vi "Copy Graph to Clipboard.vi"(8 "error in (no error)":errorcluster, 11 "Graph Data":T1={"UI References"={"Exit Ref"=refnum, "Save Ref"=refnum, "Open Ref"=refnum, "Export Ref"=refnum, "Acquire Ref"=refnum, "Configure Ref"=refnum, "Graph Ref"=refnum, "Clear Ref"=refnum, "Analyze Ref"=refnum, "Status Ref"=refnum, "Snapshot Ref"=refnum}, "User Specified"={"Hardware Configuration"={"VGC50"={"serial settings"={"port"="", "baud rate"=115200}, "device information"={"type"="", "model number"="", "serial number"="", "firmware version"="", "hardware version"=""}, "gauges"=[], "VGC"=refnum, "Backing SP"={"mode"=0, "thresholds"={"lower"=0.0, "upper"=0.0}, "on"=FALSE}, "Chamber SP"={"mode"=1, "thresholds"={"lower"=0.0, "upper"=0.0}, "on"=FALSE}}, "PTC10"={"serial settings"={"port"="GPIB0::22::INSTR", "baud rate"=115200}, "PTC10 Info"={"Manufacturer"="", "Instrument"="", "Serial Number"="", "Firmware"=""}, "VISA resource name"=""}}, "New Data Behavior"=enum."Replace", "Vacuum Graph config"={"Log/Lin"=FALSE, "Show Backing"=FALSE, "Show Chamber"=FALSE}}} {"User Specified"."Hardware Configuration"."PTC10"."serial settings"."baud rate" items=["9600"=9600, "19200"=19200, "38400"=38400, "57600"=57600, "115200"=115200]; "User Specified"."Hardware Configuration"."VGC50"."Chamber SP"."thresholds"."upper" format="%#_5p"; "User Specified"."Hardware Configuration"."VGC50"."Chamber SP"."thresholds"."lower" format="%#_5p"; "User Specified"."Hardware Configuration"."VGC50"."Chamber SP"."mode" items=["off", "on", "channel 1", "channel 2", "channel 3"]; "User Specified"."Hardware Configuration"."VGC50"."Backing SP"."thresholds"."upper" format="%#_5p"; "User Specified"."Hardware Configuration"."VGC50"."Backing SP"."thresholds"."lower" format="%#_5p"; "User Specified"."Hardware Configuration"."VGC50"."Backing SP"."mode" items=["off", "on", "channel 1", "channel 2", "channel 3"]; "User Specified"."Hardware Configuration"."VGC50"."gauges"."status" items=["data ok", "underrange", "overrange", "sensor error", "sensor off", "no sensor", "identification error", "error BPG, HPG, BCG"]; "User Specified"."Hardware Configuration"."VGC50"."gauges"."value" format="%#_4p"; "User Specified"."Hardware Configuration"."VGC50"."serial settings"."baud rate" items=["9600"=9600, "19200"=19200, "38400"=38400, "57600"=57600, "115200"=115200]}) -> (0 "error out":errorcluster)   [LabVIEW 2023]
doc: "Copies an image of the graph to the clipboard."
uses:
  controls/UI References.ctl
  controls/HW Configuration.ctl
  controls/New Data Behavior.ctl
  controls/User Specified Data.ctl
  controls/Data.ctl
  controls/VGC50.ctl
  <instrlib>/PL Inficon VGC/PL Inficon VGC.lvclass
  controls/Vac Graph Config.ctl
  controls/SRS PTC10.ctl
panel:
  # "(Scroll up to see large data cluster)"
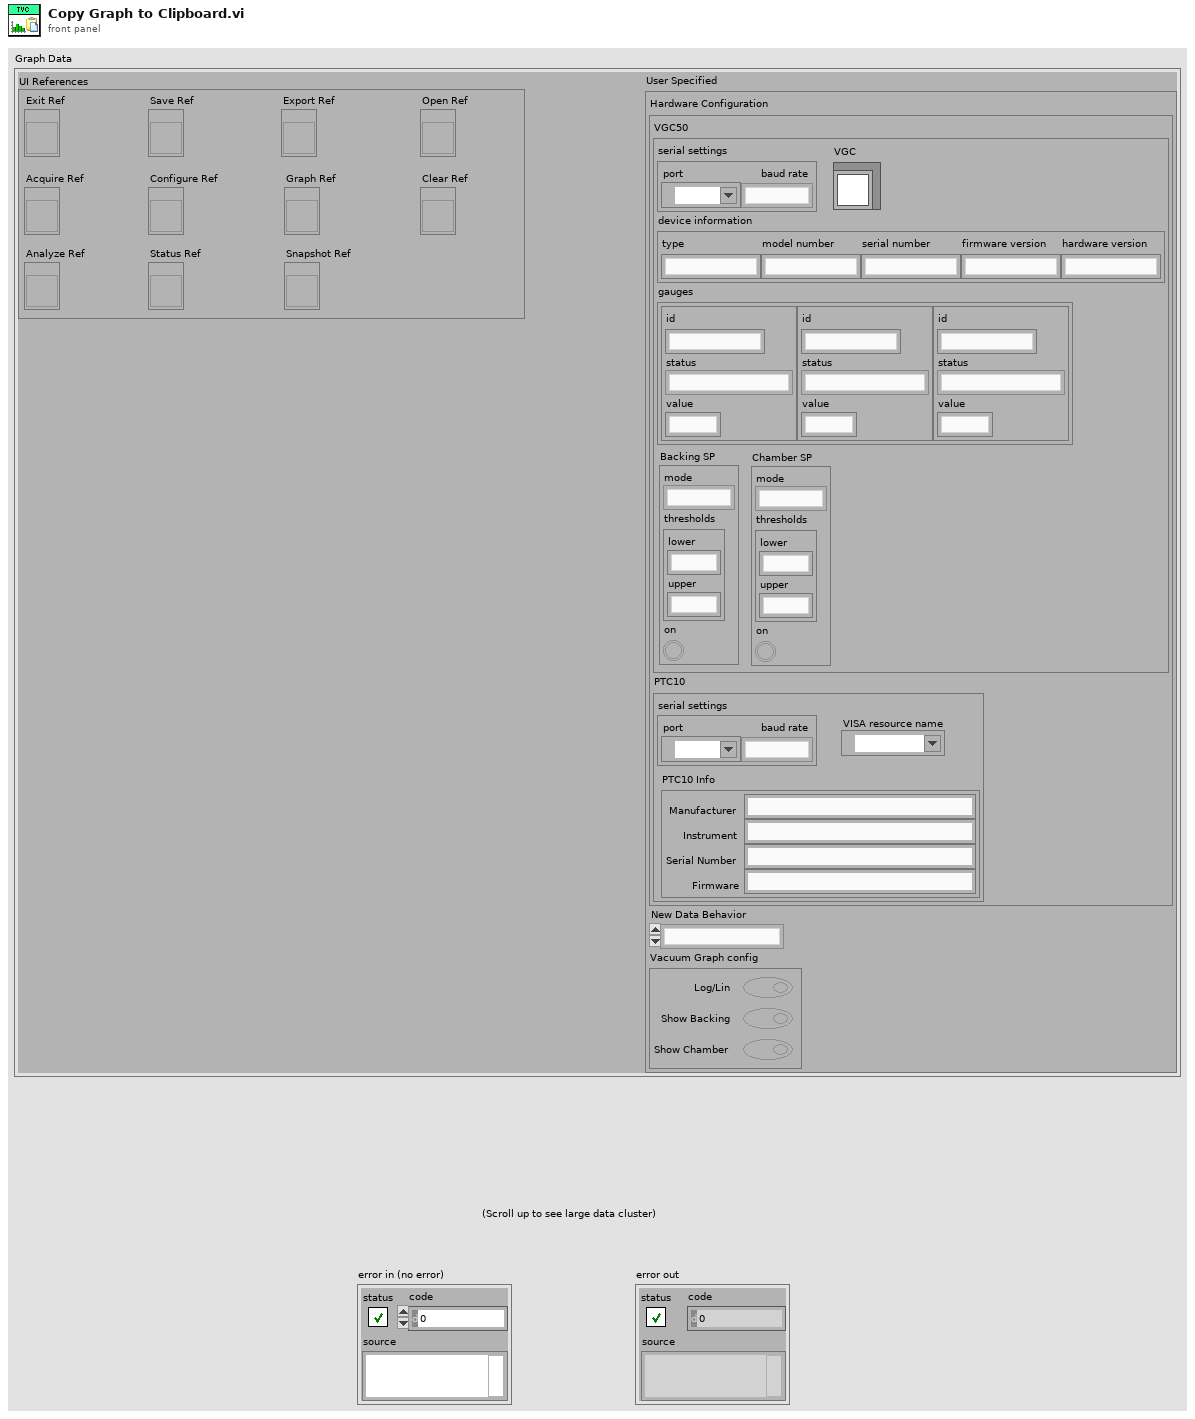
[diagram p1: front panel]
types:
  T1 = typedef "Data.ctl" = cluster{"UI References":T2, "User Specified":T3}
  T2 = typedef "UI References.ctl" = cluster{"Exit Ref":refnum<vi>, "Save Ref":refnum<vi>, "Open Ref":refnum<vi>, "Export Ref":refnum<vi>, "Acquire Ref":refnum<vi>, "Configure Ref":refnum<vi>, "Graph Ref":refnum<vi>, "Clear Ref":refnum<vi>, "Analyze Ref":refnum<vi>, "Status Ref":refnum<vi>, "Snapshot Ref":refnum<vi>}
  T3 = typedef "User Specified Data.ctl" = cluster{"Hardware Configuration":T4, "New Data Behavior":T7, "Vacuum Graph config":T8}
  T4 = typedef "HW Configuration.ctl" = cluster{"VGC50":T5, "PTC10":T6}
  T5 = typedef "VGC50.ctl" = cluster{"serial settings":cluster{"port":refnum<visa-resource-name>, "baud rate":u32}, "device information":cluster{"type":string, "model number":string, "serial number":string, "firmware version":string, "hardware version":string}, "gauges":cluster{"id":string, "status":u16, "value":dbl}[], "VGC":refnum<class "PL Inficon VGC.lvclass">, "Backing SP":cluster{"mode":u16, "thresholds":cluster{"lower":dbl, "upper":dbl}, "on":bool}, "Chamber SP":cluster{"mode":u16, "thresholds":cluster{"lower":dbl, "upper":dbl}, "on":bool}}
  T6 = typedef "SRS PTC10.ctl" = cluster{"serial settings":cluster{"port":refnum<visa-resource-name>, "baud rate":u32}, "PTC10 Info":cluster{"Manufacturer":string, "Instrument":string, "Serial Number":string, "Firmware":string}, "VISA resource name":refnum<visa-resource-name>}
  T7 = typedef "New Data Behavior.ctl" = enum16{"Replace", "Overlay", "Append"}
  T8 = typedef "Vac Graph Config.ctl" = cluster{"Log/Lin":bool, "Show Backing":bool, "Show Chamber":bool}
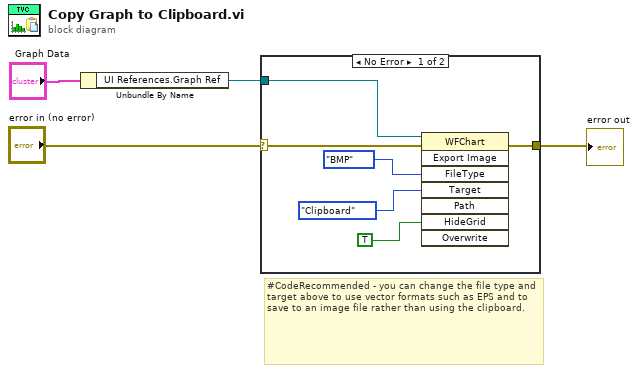
[diagram p0: block diagram]
diagram:
  # "#CodeRecommended - you can change the file type and target above to use vector formats such as EPS and to save to an image file rather than using the clipboard."
  n1 = Unbundle By Name("Graph Data") -> ("UI References.Graph Ref"=w3:refnum<vi>)
  n2 = case shown="No Error" "error in (no error)" {
    selector: "error in (no error)" -> [w5 w11]
    tunnel: w3 -> [w10 _]
    tunnel: [w6 w11] -> w2
    frame No Error {
      n3 = invoke class="WFChart" method="Export Image"(reference=w10, error in=w5, "FileType"=enum32{"BMP", "EPS", "EMF", "PICT"}."BMP" ("File Type"), "Target"=enum32{"File", "Clipboard"}."Clipboard", "HideGrid"=TRUE ("Hide Grid")) -> (error out=w6:errorcluster)  [unwired: 3 in, 7 out]
    }
    frame Error {
    }
  }
  "error out" <- w2
